vi "Init.vi"(0 "Type Name Path":map{string, map{string, path}}(c390), 4 "Rename":string, 6 "Name":string, 8 "Type":string, 9 "Project:Active Project":refnum<vi>, 10 "NI.LV.Dialog Instance":refnum<vi>) -> (3 "Script out":refnum<class "_Rename.lvclass">)   [LabVIEW 2021, in "_Rename.lvlib" / "_Rename.lvclass"]
uses:
  _Rename.lvclass
  _Rename.lvclass/_Rename.ctl
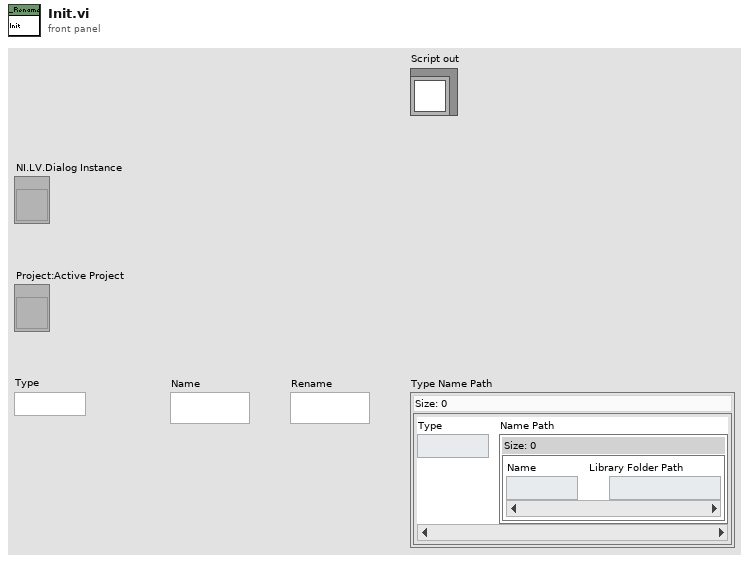
[diagram p1: front panel]
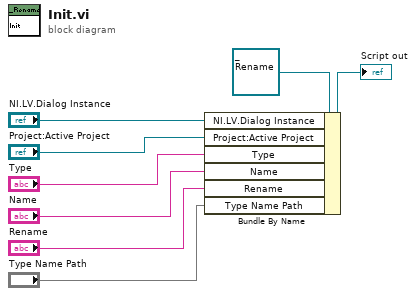
[diagram p0: block diagram]
diagram:
  n1 = Bundle By Name(cluster=refnum<class "_Rename.lvclass"> refnum ("Script out"), "NI.LV.Dialog Instance"="NI.LV.Dialog Instance", "Project:Active Project"="Project:Active Project", "Type"="Type", "Name"="Name", "Rename"="Rename", "Type Name Path"="Type Name Path") -> (→"Script out":refnum<class "_Rename.lvclass">)
